vi "PDF Protokolle gemeinsam.vi"(3 "start":bool, 4 "LIN/EPA":enum16{"LIN", "EPA", "LIN + EPA"}(ring), 5 "Pfad LIN":T11, 6 "File Names":T2, 7 "Graphs":T10, 8 "Fehler (Eingang, kein Fehler)":errorcluster, 9 "SpanComponentInfos-Cluster":T7, 10 "PDF Optionen":T8, 11 "Polynom-Ordnung":T1) -> (0 "Fehler (Ausgang)":errorcluster, 1 "EPA Context (Ausgang)":refnum<class "Context.lvclass">, 2 "Context (Ausgang)":refnum<class "Context.lvclass">)   [LabVIEW 2020, in "Linearisierung v2.lvlib" / "Protokoll.lvlib"]
uses:
  Protokoll.lvlib
  PDF_Interface/PDF Interface.lvlib
  SpanEinstellungen/SpanEinstellungen.lvlib
  Visualisierungs Elemente/Pfad-Eingabefeld.ctl
  Visualisierungs Elemente/String - Eingabefeld.ctl
  <vilib>/Simplicity AI/SAI_PDF_API/Classes/Context/Context.lvclass
  Visualisierungs Elemente/String - Ausgabefeld.ctl
  SpanEinstellungen/ComponentInfos.ctl
  SpanEinstellungen/SpanComponentInfos-Cluster.ctl
  SpanEinstellungen/PDF Optionen.ctl
  Auswahl Polynom Ordnung.ctl
  Linearisierung v2.lvlib
  PDF_Interface/PDF Interface Helper/PDFResultPictures.ctl
  PDF_Interface/PDF Interface Helper/PDF Interface Helper.lvlib
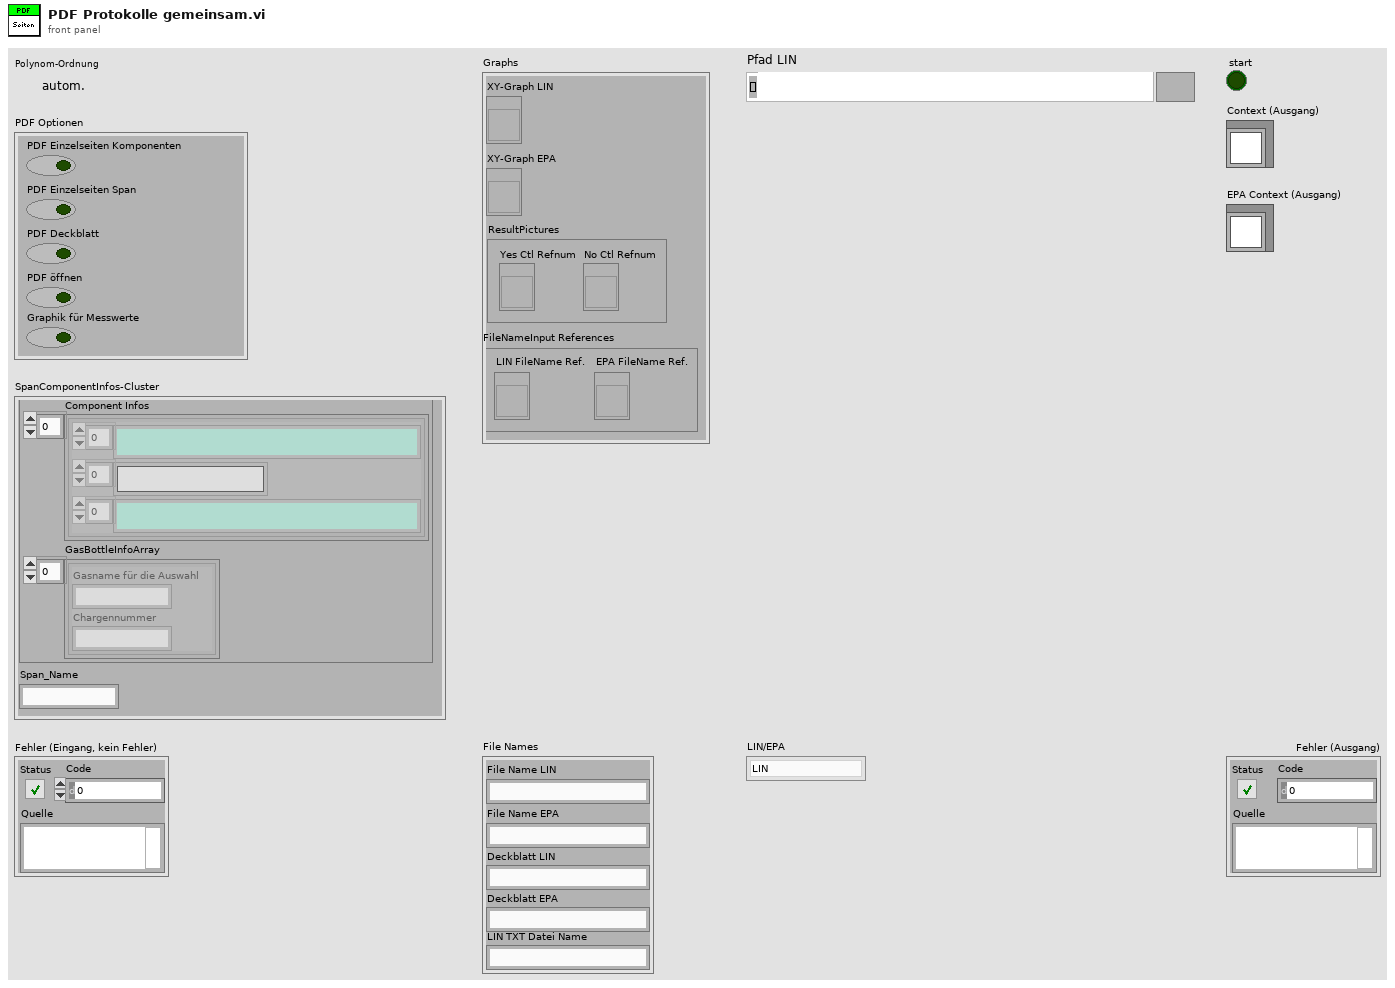
[diagram p1: front panel]
types:
  T1 = typedef "Linearisierung v2.lvlib/Auswahl Polynom Ordnung.ctl" = enum16{"autom.", "raw", "actual", "1", "2", "3", "4"}
  T2 = cluster{"File Name LIN":string, "File Name EPA":string, "Deckblatt LIN":string, "Deckblatt EPA":string, "LIN TXT Datei Name":string}
  T3 = typedef "Linearisierung v2.lvlib/SpanEinstellungen.lvlib/SpanComponentInfos-Cluster.ctl" = cluster{"SPAN Names":string[], "Component Infos":T4[], "GasBottleInfoArray":cluster{"Gasname für die Auswahl":string, "Chargennummer":string}[]}
  T4 = typedef "Linearisierung v2.lvlib/SpanEinstellungen.lvlib/ComponentInfos.ctl" = cluster{T5[], T6[], T5[]}
  T5 = typedef "String - Ausgabefeld.ctl" = string
  T6 = typedef "String - Eingabefeld.ctl" = string
  T7 = cluster{"SpanComponentInfos-Cluster":T3, "Span_Name":string}
  T8 = typedef "Linearisierung v2.lvlib/SpanEinstellungen.lvlib/PDF Optionen.ctl" = cluster{"PDF Einzelseiten Komponenten":bool, "PDF Einzelseiten Span":bool, "PDF Deckblatt":bool, "PDF öffnen":bool, "Graphik für Messwerte":bool}
  T9 = typedef "PDF Interface.lvlib/PDF Interface Helper.lvlib/PDFResultPictures.ctl" = cluster{"Yes Ctl Refnum":refnum<vi>, "No Ctl Refnum":refnum<vi>}
  T10 = cluster{"XY-Graph LIN":refnum<vi>, "XY-Graph EPA":refnum<vi>, "ResultPictures":T9, "FileNameInput References":cluster{"LIN FileName Ref.":refnum<vi>, "EPA FileName Ref.":refnum<vi>}}
  T11 = typedef "Pfad-Eingabefeld.ctl" = path
  T12 = cluster{"LIN FileName Ref.":refnum<vi>, "EPA FileName Ref.":refnum<vi>}
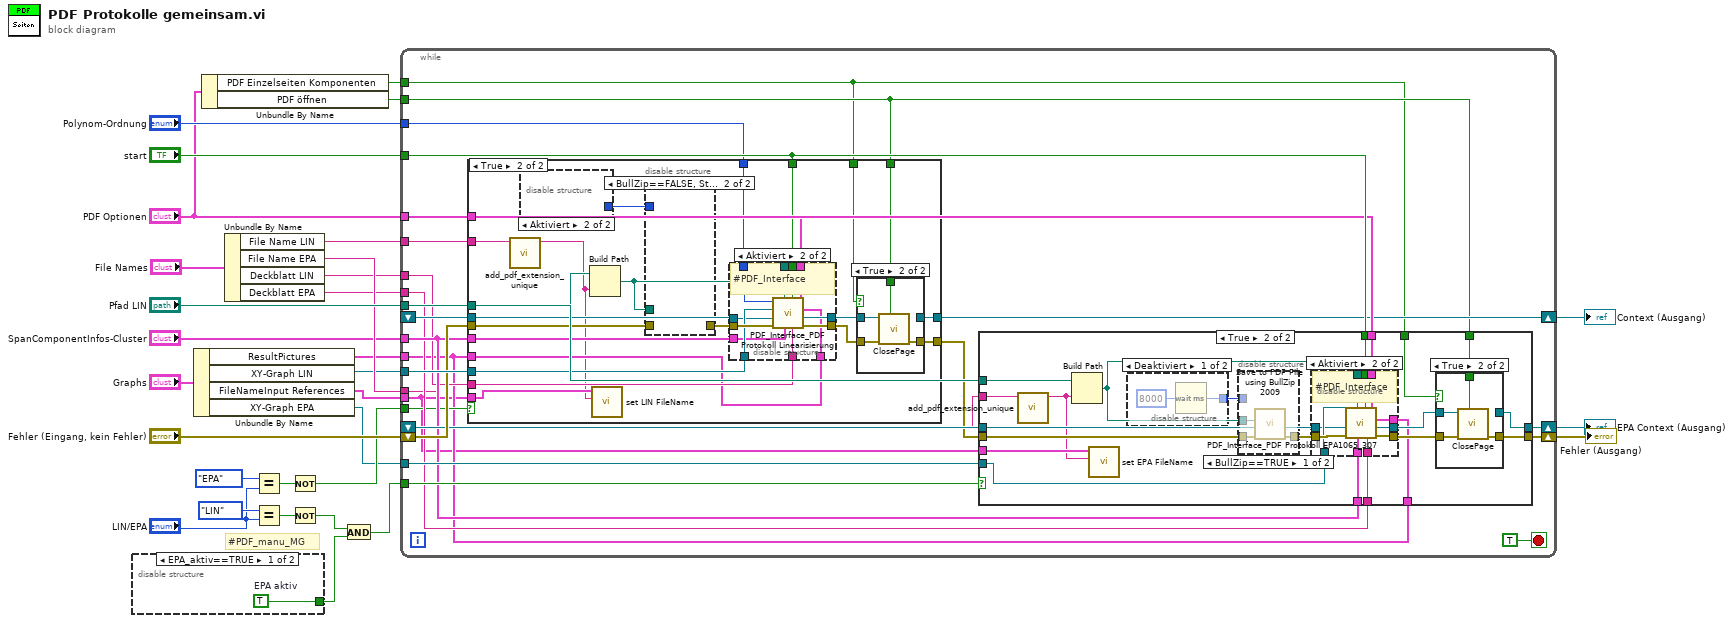
[diagram p0: block diagram]
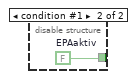
[diagram p2: hidden frame]
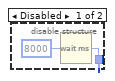
[diagram p5: hidden frame]
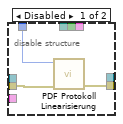
[diagram p6: hidden frame]
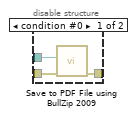
[diagram p7: hidden frame]
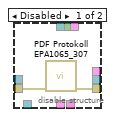
[diagram p11: hidden frame]
diagram:
  # "#PDF_manu_MG"
  n1 = disable-structure shown="EPA_aktiv==TRUE" {
    disable-tunnel: [w31 w32] -> w16
    frame condition #0 (active) {
      w31 = TRUE  # EPA aktiv
    }
    frame condition #1 {
      w32 = FALSE  # EPAaktiv
    }
  }
  n2 = Unbundle By Name("Graphs") -> ("ResultPictures"=w3:T9, "XY-Graph LIN"=w22:refnum<vi>, "FileNameInput References"=w1:T12, "XY-Graph EPA"=w2:refnum<vi>)
  n3 = Unbundle By Name("PDF Optionen") -> ("PDF Einzelseiten Komponenten"=w9:bool, "PDF öffnen"=w10:bool)
  n4 = Unbundle By Name("File Names") -> ("File Name LIN"=w25:string, "File Name EPA"=w24:string, "Deckblatt LIN"=w19:string, "Deckblatt EPA"=w18:string)
  n5 = Equal?(x=enum16{"LIN", "EPA", "LIN + EPA"}."EPA", y="LIN/EPA") -> (x = y?=w7:bool)
  n6 = Equal?(x=enum16{"LIN", "EPA", "LIN + EPA"}."LIN", y="LIN/EPA") -> (x = y?=w12:bool)
  n7 = Not(x=w7) -> (.not. x?=w4:bool)
  n8 = Not(x=w12) -> (.not. x?=w11:bool)
  n9 = And(x=w11, y=w16) -> (x .and. y?=w17:bool)
  n10 = while {
    tunnel: w22 -> [w57]
    tunnel: "Pfad LIN" -> [w55]
    tunnel: w24 -> [w33]
    tunnel: w17 -> [w54]
    tunnel: w25 -> [w53]
    tunnel: w2 -> [w49]
    tunnel: "start" -> [w48]
    shift-right: [w52] -> w28
    shift-left: "Fehler (Eingang, kein Fehler)" -> [w56]
    shift-right: [w39] -> w27
    shift-left: _ -> [w50]
    shift-right: [w51] -> w26
    shift-left: _ -> [w46]
    tunnel: "SpanComponentInfos-Cluster" -> [w45]
    tunnel: "PDF Optionen" -> [w41]
    tunnel: w19 -> [w44]
    tunnel: w18 -> [w43]
    tunnel: "Polynom-Ordnung" -> [w42]
    tunnel: w10 -> [w38]
    tunnel: w9 -> [w37]
    tunnel: w4 -> [w36]
    tunnel: w3 -> [w35]
    tunnel: w1 -> [w34]
    stop <- TRUE stop-if-true
    n11 = case shown="True" w36 {
      tunnel: w57 -> [_ w81]
      tunnel: w56 -> [w58 w79]
      tunnel: w55 -> [_ w78]
      tunnel: w53 -> [_ w76]
      tunnel: w50 -> [w59 w75]
      tunnel: w48 -> [_ w73]
      tunnel: w45 -> [_ w72]
      tunnel: w44 -> [_ w71]
      tunnel: w42 -> [_ w70]
      tunnel: w41 -> [_ w69]
      tunnel: [w58 w66] -> w40
      tunnel: [w59 w65] -> w39
      tunnel: w38 -> [_ w64]
      tunnel: w37 -> [_ w63]
      tunnel: w35 -> [_ w62]
      tunnel: w34 -> [_ w61]
      frame False {
      }
      frame True {
        n12 = call "add_pdf_extension_unique.vi"("PDF File Name in"=w76) -> ("PDF File Name out"=w60:string)  [unwired: 10 in]
        n13 = disable-structure shown="Aktiviert" {
          disable-tunnel: [w88 _] -> w74
          frame Disabled {
            n14 = Wait (ms)(milliseconds to wait=u32 8000 ("Zu wartende ms")) -> (millisecond timer value=w88:u32)
          }
          frame Enabled {
          }
        }
        n15 = Build Path(base path=w78, name or relative path=w60) -> (appended path=w80:path)
        n16 = call "set LIN FileName.vi"("File Name LIN"=w60, "FileNameInput References"=w61) -> ()  [unwired: 10 in]
        n17 = disable-structure shown="BullZip==FALSE, Standard" {
          disable-tunnel: w80 -> [w107 _]
          disable-tunnel: [w106 _] -> w77
          disable-tunnel: w79 -> [w105 _]
          disable-tunnel: w74 -> [_ _]
          frame condition #0 {
            n18 = call "Save to PDF File using BullZip 2009.vi"("error in"=w105, "Save PDF File Path"=w107) -> ("error out"=w106:errorcluster)  [unwired: 9 in]
          }
          frame condition #1 (active) {
          }
        }
        n19 = disable-structure shown="Aktiviert" {
          disable-tunnel: w77 -> [w92 w104]
          disable-tunnel: [w91 w103] -> w67
          disable-tunnel: w70 -> [w90 w102]
          disable-tunnel: w80 -> [_ w101]
          disable-tunnel: w81 -> [_ w100]
          disable-tunnel: [_ w99] -> w68
          disable-tunnel: w75 -> [_ w98]
          disable-tunnel: w73 -> [_ w97]
          disable-tunnel: w72 -> [_ w96]
          disable-tunnel: w69 -> [_ w95]
          disable-tunnel: w71 -> [_ w94]
          disable-tunnel: w62 -> [_ w93]
          frame Disabled {
            n20 = call "PDF Protokoll Linearisierung.vi"("error in (no error)"=w92, "Polynom-Ordnung"=w90) -> ("error out"=w91:errorcluster)  [unwired: 9 in]
          }
          frame Enabled {
            # "#PDF_Interface"
            n21 = call "PDF_Interface_PDF Protokoll Linearisierung.vi"("ResultPictures"=w93, "PDF Optionen"=w95, "Deckblatt_Name"=w94, "start"=w97, "SpanComponentInfos-Cluster"=w96, "Save PDF File Path"=w101, "error in (no error)"=w104, "Context (Eingang)"=w98, "XY-Graph LIN"=w100, "Polynom-Ordnung"=w102) -> ("error out"=w103:errorcluster, "Context (Ausgang)"=w99:refnum<class "Context.lvclass">)
          }
        }
        n22 = case shown="True" w63 {
          tunnel: w67 -> [w83 w87]
          tunnel: w64 -> [_ w86]
          tunnel: w68 -> [w82 w85]
          tunnel: [w83 w84] -> w66
          tunnel: [w82 _] -> w65
          frame False {
          }
          frame True {
            n23 = call "ClosePage.vi"("popup viewer"=w86, "Fehler (Eingang, kein Fehler)"=w87, "Context (Eingang)"=w85) -> ("Fehler (Ausgang)"=w84:errorcluster)  [unwired: 8 in]
          }
        }
      }
    }
    n24 = case shown="True" w54 {
      tunnel: w55 -> [_ w129]
      tunnel: w33 -> [_ w111]
      tunnel: [w109 w118] -> w52
      tunnel: w40 -> [w109 w127]
      tunnel: [w108 w114] -> w51
      tunnel: w49 -> [_ w125]
      tunnel: w48 -> [_ w124]
      tunnel: w46 -> [w108 w123]
      tunnel: w45 -> [_ w122]
      tunnel: w41 -> [_ w121]
      tunnel: w43 -> [_ w120]
      tunnel: w37 -> [_ w116]
      tunnel: w38 -> [_ w115]
      tunnel: w35 -> [_ w113]
      tunnel: w34 -> [_ w112]
      frame False {
      }
      frame True {
        n25 = call "add_pdf_extension_unique.vi"("PDF File Name in"=w111) -> ("PDF File Name out"=w110:string)  [unwired: 10 in]
        n26 = Build Path(base path=w129, name or relative path=w110) -> (appended path=w126:path)
        n27 = call "set EPA FileName.vi"("File Name EPA"=w110, "FileNameInput References"=w112) -> ()  [unwired: 10 in]
        n28 = disable-structure shown="Deaktiviert" {
          disable-tunnel: [w137 _] -> w128
          frame Disabled {
            n29 = Wait (ms)(milliseconds to wait=u32 8000 ("Zu wartende ms")) -> (millisecond timer value=w137:u32)
          }
          frame Enabled {
          }
        }
        n30 = disable-structure shown="BullZip==TRUE" {
          disable-tunnel: [w154 _] -> w130
          disable-tunnel: w126 -> [w153 _]
          disable-tunnel: w128 -> [_ _]
          disable-tunnel: w127 -> [w152 _]
          frame condition #0 {
            n31 = call "Save to PDF File using BullZip 2009.vi"("error in"=w152, "Save PDF File Path"=w153) -> ("error out"=w154:errorcluster)  [unwired: 9 in]
          }
          frame condition #1 (active) {
          }
        }
        n32 = disable-structure shown="Aktiviert" {
          disable-tunnel: w130 -> [w140 w151]
          disable-tunnel: [w139 w150] -> w119
          disable-tunnel: w126 -> [_ w149]
          disable-tunnel: w125 -> [_ w148]
          disable-tunnel: [_ w147] -> w117
          disable-tunnel: w124 -> [_ w146]
          disable-tunnel: w123 -> [_ w145]
          disable-tunnel: w122 -> [_ w144]
          disable-tunnel: w121 -> [_ w143]
          disable-tunnel: w120 -> [_ w142]
          disable-tunnel: w113 -> [_ w141]
          frame Disabled {
            n33 = call "PDF Protokoll EPA1065_307.vi"("error in (no error)"=w140) -> ("error out"=w139:errorcluster)  [unwired: 10 in]
          }
          frame Enabled {
            # "#PDF_Interface"
            n34 = call "PDF_Interface_PDF Protokoll EPA1065_307.vi"("ResultPictures"=w141, "PDF Optinen"=w143, "Deckblatt_Name"=w142, "start"=w146, "SpanComponentInfos-Cluster"=w144, "Save PDF File Path"=w149, "error in (no error)"=w151, "Context (Eingang)"=w145, "XY-Graph EPA"=w148) -> ("error out"=w150:errorcluster, "Context (Ausgang)"=w147:refnum<class "Context.lvclass">)  [unwired: 1 in]
          }
        }
        n35 = case shown="True" w116 {
          tunnel: w119 -> [w132 w136]
          tunnel: [w132 w135] -> w118
          tunnel: w117 -> [w131 w134]
          tunnel: w115 -> [_ w133]
          tunnel: [w131 _] -> w114
          frame False {
          }
          frame True {
            n36 = call "ClosePage.vi"("popup viewer"=w133, "Fehler (Eingang, kein Fehler)"=w136, "Context (Eingang)"=w134) -> ("Fehler (Ausgang)"=w135:errorcluster)  [unwired: 8 in]
          }
        }
      }
    }
  }
  "Fehler (Ausgang)" <- w28
  "Context (Ausgang)" <- w27
  "EPA Context (Ausgang)" <- w26
